vi "BotoesControle.vi"() -> ()   [LabVIEW 2018]
panel:
  in  "Botao6":bool
  in  "Botao5":bool
  in  "Botao4":bool
  in  "Botao2":bool
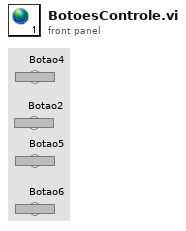
[diagram p1: front panel]
diagram:
